vi "Allowed Commands.vi"() -> (2 "Allowed Commands":string[](array[string]))   [LabVIEW 2020]
doc: "Builds the allowed commands array from the enum and additional commands."
uses:
  Command Enum.ctl
  <vilib>/Utility/Data Type/NI_Data Type.lvlib
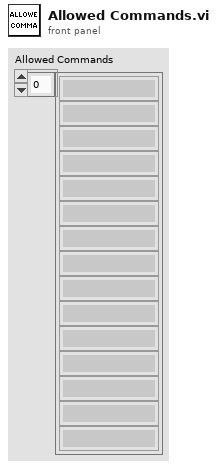
[diagram p1: front panel]
types:
  T1 = typedef "Command Enum.ctl" = enum16{"Invalid", "Run", "Set", "Open", "Read", "Remove"}
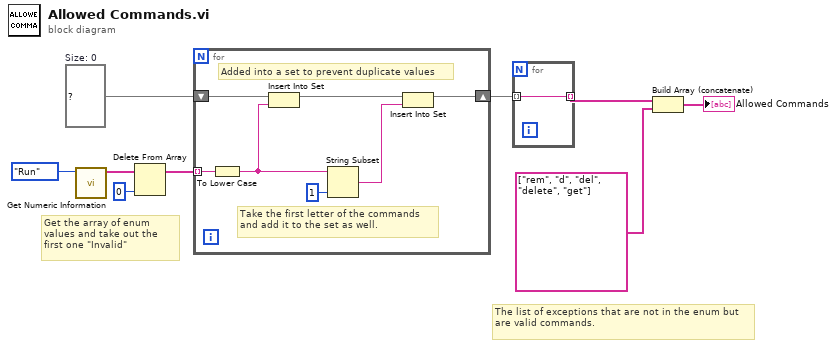
[diagram p0: block diagram]
diagram:
  w8 = set{string} {}  # Size: 0
  # "The list of exceptions that are not in the enum but are valid commands."
  # "Get the array of enum values and take out the first one \"Invalid\""
  n1 = call <vilib>:"Get Numeric Information.vi"("variant"=Command_Enum."Run" ("Command")) -> ("enum names"=w7:string[])  [unwired: 7 in, 3 out]
  n2 = Delete From Array(array=w7, index=0) -> (array with subset deleted=w6:string[])  [unwired: 1 in, 1 out]
  n3 = for {
    shift-right: [w10] -> w4
    shift-left: w8 -> [w16]
    tunnel: w6 -> [w15] mode=indexing
    # "Take the first letter of the commands \nand add it to the set as well."
    # "Added into a set to prevent duplicate values"
    n4 = To Lower Case(string=w15) -> (all lower case string=w13:string)
    n5 = Insert Into Set(10:w13, 11:w16) -> (3:w14:set{string})  [unwired: 1 out]
    n6 = String Subset(string=w13, length (rest)=1 ("length (rest)")) -> (substring=w11:string)  [unwired: 1 in]
    n7 = Insert Into Set(10:w11, 11:w14) -> (3:w10:set{string})  [unwired: 1 out]
  }
  n8 = for {
    tunnel: [w17] -> w3 mode=indexing
    tunnel: w4 -> [w17] mode=indexing
  }
  n9 = Build Array (concatenate)(w3, string[] ["rem", "d", "del", "delete", "get"] ("array")) -> (→"Allowed Commands":string[])
